vi "Send to Open Instruments.vi"(7 "Instrument Names":string[](array[string]), 8 "error in (no error)":errorcluster, 9 "Message Data":variant, 10 "Command":string=": Exit", 11 "Master":refnum<queue>) -> (0 "error out":errorcluster)   [LabVIEW 2014, in "MeasurementControl Message Queue.lvlib"]
uses:
  Message Cluster.ctl
  MeasurementControl Message Queue.lvlib
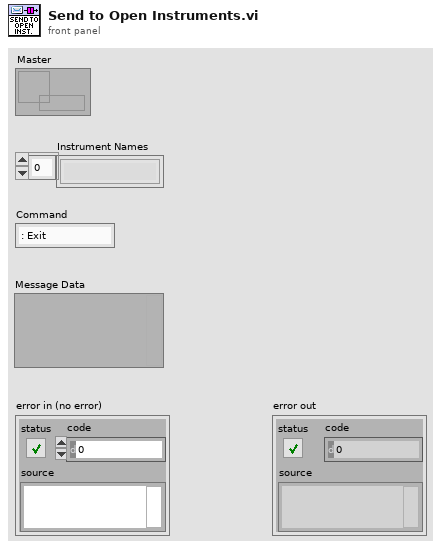
[diagram p1: front panel]
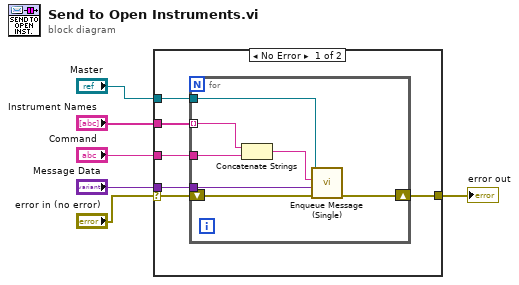
[diagram p0: block diagram]
diagram:
  n1 = case shown="No Error" "error in (no error)" {
    selector: "error in (no error)" -> [w9 w20]
    tunnel: "Instrument Names" -> [w12 _]
    tunnel: "Master" -> [w11 _]
    tunnel: [w10 w20] -> w3
    tunnel: "Command" -> [w8 _]
    tunnel: "Message Data" -> [w7 _]
    frame No Error {
      n2 = for {
        tunnel: w12 -> [w19] mode=indexing
        tunnel: w11 -> [w18]
        shift-right: [w16] -> w10
        shift-left: w9 -> [w15]
        tunnel: w8 -> [w14]
        tunnel: w7 -> [w13]
        n3 = Concatenate Strings(w19, w14) -> (w17:string)
        n4 = call "Enqueue Message (Single).vi"("error in (no error)"=w15, "Message Data"=w13, "Message"=w17, "Message Queue"=w18) -> ("error out"=w16:errorcluster)  [unwired: 6 in, 1 out]
      }
    }
    frame Error {
    }
  }
  "error out" <- w3
